vi "ex1.vi"() -> ()   [LabVIEW 2022 SP3]
uses:
  ex1_cluster.ctl
panel:
  out "error out":errorcluster
  in  "error in":errorcluster
  out "Total area result":i32
  in  "Cluster":T1
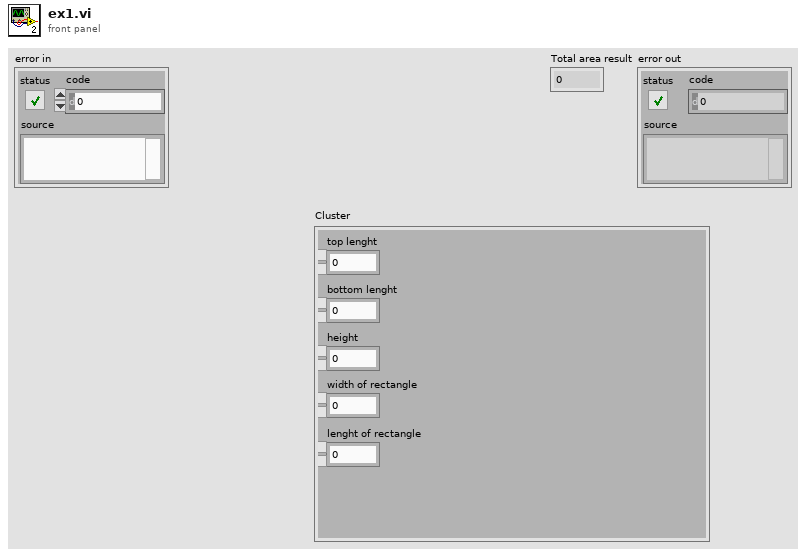
[diagram p1: front panel]
types:
  T1 = typedef "ex1_cluster.ctl" = cluster{"top lenght ":dbl, "bottom lenght":dbl, "height":dbl, "width of rectangle ":dbl, "lenght of rectangle ":dbl}
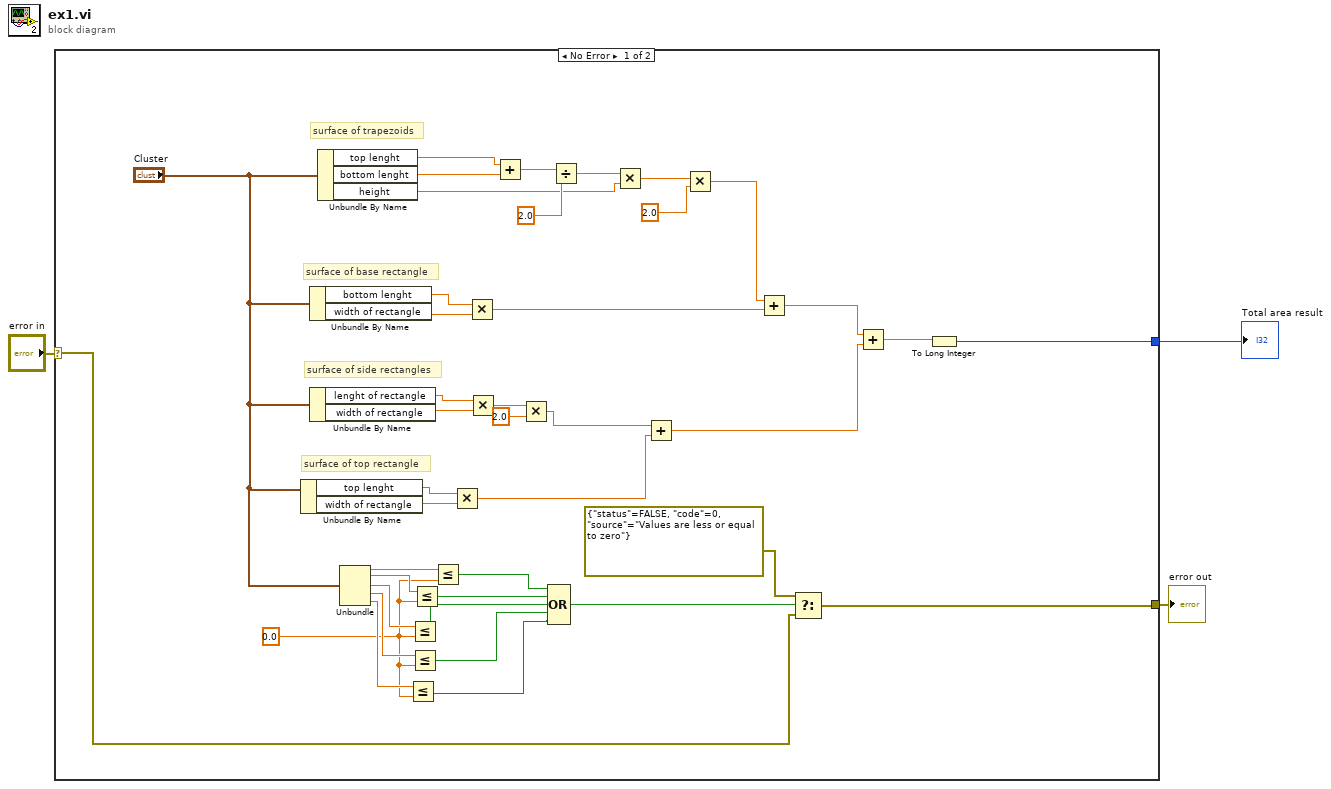
[diagram p0: block diagram]
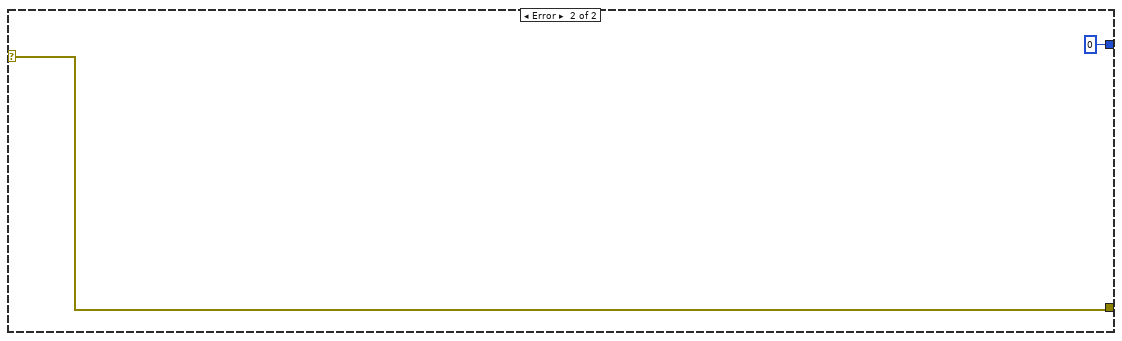
[diagram p2: hidden frame]
diagram:
  n1 = case shown="No Error" "error in" {
    selector: "error in" -> [w6 w45]
    tunnel: [w5 0] -> w2
    tunnel: [w4 w45] -> w1
    frame No Error {
      w14 = 0.0 ("y")
      # "surface of top rectangle"
      # "surface of side rectangles"
      # "surface of base rectangle"
      # "surface of trapezoids"
      n2 = Unbundle By Name("Cluster") -> ("top lenght"=w29:dbl, "width of rectangle"=w28:dbl)
      n3 = Unbundle By Name("Cluster") -> ("bottom lenght"=w35:dbl, "width of rectangle"=w34:dbl)
      n4 = Unbundle By Name("Cluster") -> ("lenght of rectangle"=w33:dbl, "width of rectangle"=w32:dbl)
      n5 = Unbundle By Name("Cluster") -> ("top lenght"=w42:dbl, "bottom lenght"=w43:dbl, "height"=w38:dbl)
      n6 = Unbundle("Cluster") -> ("top lenght"=w19:dbl, "bottom lenght"=w18:dbl, "height"=w17:dbl, "width of rectangle"=w16:dbl, "lenght of rectangle"=w15:dbl)
      n7 = Less Or Equal?(x=w15, y=w14) -> (x <= y?=w9:bool)
      n8 = Less Or Equal?(x=w17, y=w14) -> (x <= y?=w11:bool)
      n9 = Less Or Equal?(x=w16, y=w14) -> (x <= y?=w10:bool)
      n10 = Less Or Equal?(x=w18, y=w14) -> (x <= y?=w12:bool)
      n11 = Less Or Equal?(x=w19, y=w14) -> (x <= y?=w13:bool)
      n12 = Multiply(x=w29, y=w28) -> (x*y=w24:dbl)
      n13 = Multiply(x=w35, y=w34) -> (x*y=w26:dbl)
      n14 = Multiply(x=w33, y=w32) -> (x*y=w31:dbl)
      n15 = Add(x=w42, y=w43) -> (x+y=w40:dbl)
      n16 = Multiply(x=w31, y=2.0) -> (x*y=w25:dbl)
      n17 = Compound Arithmetic op=OR(w13, w12, w11, w10, w9) -> (w8:bool)
      n18 = Divide(x=w40, y=2.0) -> (x/y=w39:dbl)
      n19 = Multiply(x=w39, y=w38) -> (x*y=w36:dbl)
      n20 = Add(x=w25, y=w24) -> (x+y=w22:dbl)
      n21 = Multiply(x=w36, y=2.0) -> (x*y=w27:dbl)
      n22 = Add(x=w27, y=w26) -> (x+y=w23:dbl)
      n23 = Select(t=errorcluster {"status"=FALSE, "code"=0, "source"="Values are less or equal to zero"} ("error constant"), s=w8, f=w6) -> (s? t:f=w4:errorcluster)
      n24 = Add(x=w23, y=w22) -> (x+y=w21:dbl)
      n25 = To Long Integer(number=w21) -> (32bit integer=w5:i32)
    }
    frame Error {
    }
  }
  "Total area result" <- w2
  "error out" <- w1
